vi "反控参数设置.vi"(8 "value time":timestamp, 9 "value float":sgl, 10 "设置参数":T2(ring)=enum."CODMn", 11 "设置类型":T1(ring)=enum."i13002") -> ()   [LabVIEW 2016]
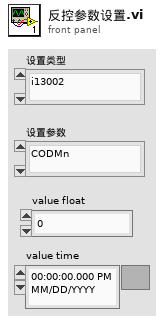
[diagram p1: front panel]
types:
  T1 = enum16{"i13001", "i13002", "i13003", "i13004", "i13005", "i13006", "i13007", "i13008", "i13009", "i13010", "i13011", "i13012", "i13013", "i13014", "i13015", "i13016", "i13017", "i13101", "i13102", "i13103", "i13104", "i13105", "i13106", "i13107", "i13108", "i13109", "i13110"}
  T2 = enum16{"", "CODMn", "PH", "氨氮", "总氮", "总磷", "CODCr", "电导率", "水温", "溶解氧", "浊度", "叶绿素", "藻密度", "ORP"}
  T3 = cluster{"status":bool, "代码":u16, "source":string}
  T4 = cluster{"测量量程":dbl, "测量精度":dbl, "测量间隔":dbl, "消解温度":dbl, "消解时长":dbl, "空白校准时间":timestamp, "曲线截距":dbl, "曲线斜率":dbl, "测量检出限":dbl, "测量信号值":dbl, "线性相关系数":dbl, "二次多项式系数":dbl, "标样校准时间":timestamp, "稀释倍数":dbl, "三项式系数":dbl, "空白标定系数":dbl, "量程系数":dbl, "F0/ORPA":dbl, "F1/ORPB":dbl, "F2/ORPK":dbl, "F3":dbl, "F4":dbl, "F5":dbl, "F6":dbl, "F7":dbl, "X0/滴定数":dbl, "量程":dbl}
  T5 = cluster{"测量量程":dbl, "测量精度":dbl, "测量间隔":dbl, "消解温度":dbl, "消解时长":dbl, "空白校准时间":timestamp, "曲线截距":dbl, "曲线斜率":dbl, "测量检出限":dbl, "测量信号值":dbl, "线性相关系数":dbl, "二次多项式系数":dbl, "标样校准时间":timestamp, "单位":u16}
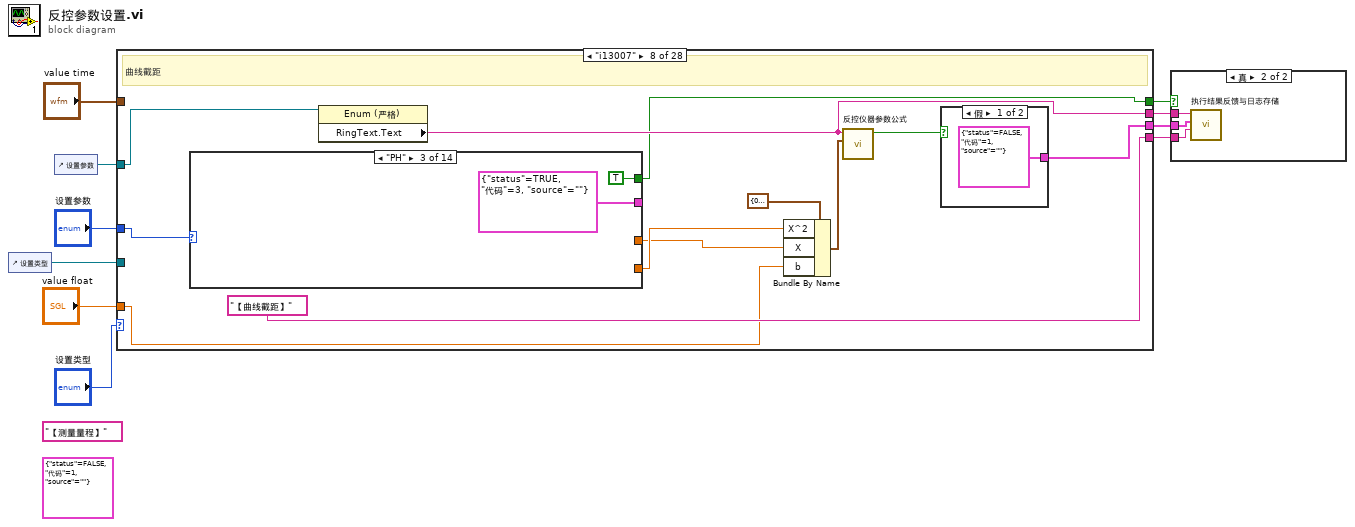
[diagram p0: block diagram]
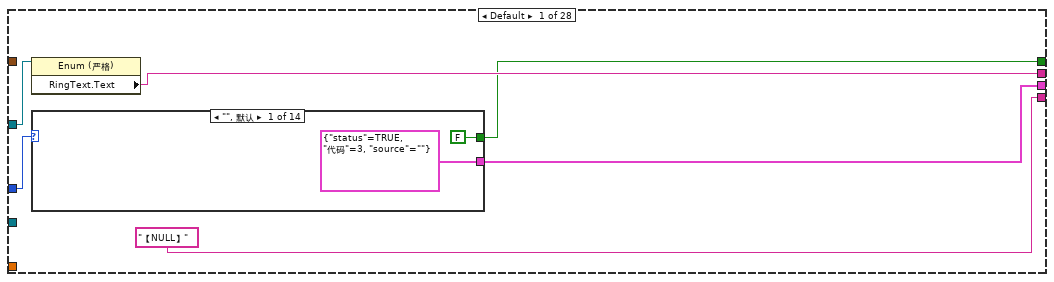
[diagram p3: hidden frame]
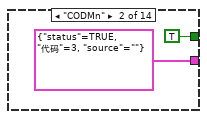
[diagram p4: hidden frame]
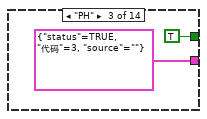
[diagram p5: hidden frame]
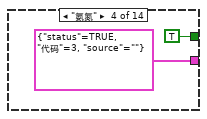
[diagram p6: hidden frame]
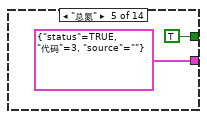
[diagram p7: hidden frame]
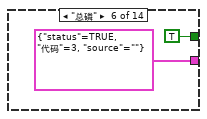
[diagram p8: hidden frame]
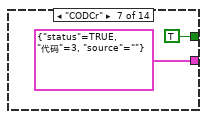
[diagram p9: hidden frame]
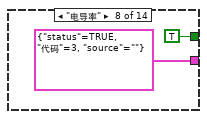
[diagram p10: hidden frame]
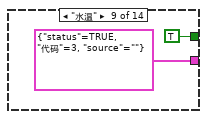
[diagram p11: hidden frame]
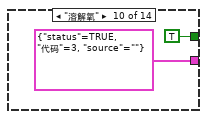
[diagram p12: hidden frame]
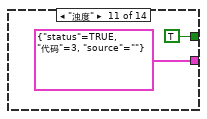
[diagram p13: hidden frame]
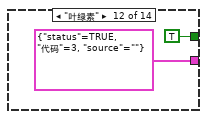
[diagram p14: hidden frame]
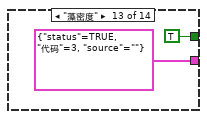
[diagram p15: hidden frame]
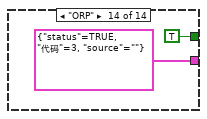
[diagram p16: hidden frame]
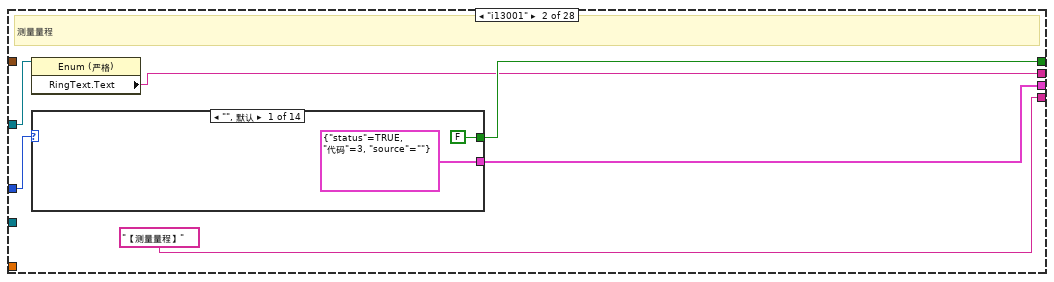
[diagram p17: hidden frame]
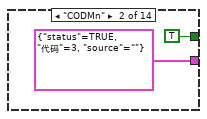
[diagram p18: hidden frame]
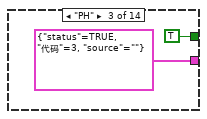
[diagram p19: hidden frame]
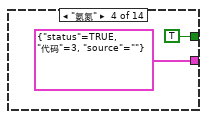
[diagram p20: hidden frame]
diagram:
  (unwired) T3 {"status"=FALSE, "代码"=1, "source"=""} ("error out")
  (unwired) "【测量量程】" ("日志信息")
  n1 = control-ref of="设置类型"() -> (w1:refnum<vi>)
  n2 = control-ref of="设置参数"() -> (w7:refnum<vi>)
  n3 = case shown="\"i13007\"" "设置类型" {
    tunnel: "设置参数" -> [w16 w50 w83 w114 w150 w193 w233 w270 w326 w381 w416 w452 w491 w540 w574 w608 w642 w676 w710 w744 w778 w816 w846 w880 w914 w948 w982 w1016]
    tunnel: [w12 w49 w80 w116 w152 w196 w236 w269 w327 w384 w418 w450 w494 w543 w577 w611 w645 w679 w713 w747 w781 w813 w849 w883 w917 w951 w985 w1019] -> w8
    tunnel: w7 -> [w15 w46 w84 w113 w154 w194 w234 w277 w334 w382 w415 w453 w492 w541 w575 w609 w643 w677 w711 w745 w779 w817 w847 w881 w915 w949 w983 w1017]
    tunnel: [w14 w45 w82 w118 w149 w190 w238 w273 w328 w386 w420 w454 w485 w545 w579 w613 w647 w681 w715 w749 w783 w815 w851 w885 w919 w953 w987 w1021] -> w6
    tunnel: ["【NULL】" ("日志信息") "【测量量程】" ("日志信息") "【测量精度】" ("日志信息") "【测量间隔】" ("日志信息") "【消解温度】" ("日志信息") "【消解时间】" ("日志信息") "【空白校准时间】" ("日志信息") "【曲线截距】" ("日志信息") "【曲线斜率】" ("日志信息") "【测量检出限】" ("日志信息") "【测量信号值】" ("日志信息") "【线性相关系数】" ("日志信息") "【二次项系数】" ("日志信息") "【标样校准时间】" ("日志信息") "【稀释倍数】" ("日志信息") "【三项式系数】" ("日志信息") "【空白标定系数】" ("日志信息") "【量程系数】" ("日志信息") "【F0/ORPA】" ("日志信息") "【F1/ORPB】" ("日志信息") "【F2/ORPK】" ("日志信息") "【F3】" ("日志信息") "【F4】" ("日志信息") "【F5】" ("日志信息") "【F6】" ("日志信息") "【F7】" ("日志信息") "【X0/滴定数】" ("日志信息") "【量程】" ("日志信息")] -> w5
    tunnel: [w13 w47 w81 w117 w153 w197 w237 w271 w330 w385 w419 w451 w487 w544 w578 w612 w646 w680 w714 w748 w782 w814 w850 w884 w918 w952 w986 w1020] -> w4
    tunnel: "value float" -> [_ _ _ _ w148 w192 _ w274 w329 _ _ _ w486 _ _ _ _ _ _ _ _ _ _ _ _ _ _ _]
    tunnel: "value time" -> [_ _ _ _ _ _ _ _ _ _ _ _ _ _ _ _ _ _ _ _ _ _ _ _ _ _ _ _]
    tunnel: w1 -> [_ _ _ _ w147 w191 _ _ _ _ _ _ _ _ _ _ _ _ _ _ _ _ _ _ _ _ _ _]
    frame Default {
      n4 = property class="Enum (严格)"(reference=w15) -> ("RingText.Text"=w14:string)  [unwired: 1 in, 2 out]
      n5 = case shown="\"\", 默认" w16 {
        tunnel: [FALSE TRUE TRUE TRUE TRUE TRUE TRUE TRUE TRUE TRUE TRUE TRUE TRUE TRUE] -> w12
        tunnel: [T3 {"status"=TRUE, "代码"=3, "source"=""} ("error out") T3 {"status"=TRUE, "代码"=3, "source"=""} ("error out") T3 {"status"=TRUE, "代码"=3, "source"=""} ("error out") T3 {"status"=TRUE, "代码"=3, "source"=""} ("error out") T3 {"status"=TRUE, "代码"=3, "source"=""} ("error out") T3 {"status"=TRUE, "代码"=3, "source"=""} ("error out") T3 {"status"=TRUE, "代码"=3, "source"=""} ("error out") T3 {"status"=TRUE, "代码"=3, "source"=""} ("error out") T3 {"status"=TRUE, "代码"=3, "source"=""} ("error out") T3 {"status"=TRUE, "代码"=3, "source"=""} ("error out") T3 {"status"=TRUE, "代码"=3, "source"=""} ("error out") T3 {"status"=TRUE, "代码"=3, "source"=""} ("error out") T3 {"status"=TRUE, "代码"=3, "source"=""} ("error out") T3 {"status"=TRUE, "代码"=3, "source"=""} ("error out")] -> w13
        frame "", Default {
        }
        frame "CODMn" {
        }
        frame "PH" {
        }
        frame "氨氮" {
        }
        frame "总氮" {
        }
        frame "总磷" {
        }
        frame "CODCr" {
        }
        frame "电导率" {
        }
        frame "水温" {
        }
        frame "溶解氧" {
        }
        frame "浊度" {
        }
        frame "叶绿素" {
        }
        frame "藻密度" {
        }
        frame "ORP" {
        }
      }
    }
    frame "i13001" {
      # "测量量程"
      n6 = property class="Enum (严格)"(reference=w46) -> ("RingText.Text"=w45:string)  [unwired: 1 in, 2 out]
      n7 = case shown="\"\", 默认" w50 {
        tunnel: [FALSE TRUE TRUE TRUE TRUE TRUE TRUE TRUE TRUE TRUE TRUE TRUE TRUE TRUE] -> w49
        tunnel: [T3 {"status"=TRUE, "代码"=3, "source"=""} ("error out") T3 {"status"=TRUE, "代码"=3, "source"=""} ("error out") T3 {"status"=TRUE, "代码"=3, "source"=""} ("error out") T3 {"status"=TRUE, "代码"=3, "source"=""} ("error out") T3 {"status"=TRUE, "代码"=3, "source"=""} ("error out") T3 {"status"=TRUE, "代码"=3, "source"=""} ("error out") T3 {"status"=TRUE, "代码"=3, "source"=""} ("error out") T3 {"status"=TRUE, "代码"=3, "source"=""} ("error out") T3 {"status"=TRUE, "代码"=3, "source"=""} ("error out") T3 {"status"=TRUE, "代码"=3, "source"=""} ("error out") T3 {"status"=TRUE, "代码"=3, "source"=""} ("error out") T3 {"status"=TRUE, "代码"=3, "source"=""} ("error out") T3 {"status"=TRUE, "代码"=3, "source"=""} ("error out") T3 {"status"=TRUE, "代码"=3, "source"=""} ("error out")] -> w47
        frame "", Default {
        }
        frame "CODMn" {
        }
        frame "PH" {
        }
        frame "氨氮" {
        }
        frame "总氮" {
        }
        frame "总磷" {
        }
        frame "CODCr" {
        }
        frame "电导率" {
        }
        frame "水温" {
        }
        frame "溶解氧" {
        }
        frame "浊度" {
        }
        frame "叶绿素" {
        }
        frame "藻密度" {
        }
        frame "ORP" {
        }
      }
    }
    frame "i13002" {
      # "测量精度"
      n8 = property class="Enum (严格)"(reference=w84) -> ("RingText.Text"=w82:string)  [unwired: 1 in, 2 out]
      n9 = case shown="\"\", 默认" w83 {
        tunnel: [FALSE TRUE TRUE TRUE TRUE TRUE TRUE TRUE TRUE TRUE TRUE TRUE TRUE TRUE] -> w80
        tunnel: [T3 {"status"=TRUE, "代码"=3, "source"=""} ("error out") T3 {"status"=TRUE, "代码"=3, "source"=""} ("error out") T3 {"status"=TRUE, "代码"=3, "source"=""} ("error out") T3 {"status"=TRUE, "代码"=3, "source"=""} ("error out") T3 {"status"=TRUE, "代码"=3, "source"=""} ("error out") T3 {"status"=TRUE, "代码"=3, "source"=""} ("error out") T3 {"status"=TRUE, "代码"=3, "source"=""} ("error out") T3 {"status"=TRUE, "代码"=3, "source"=""} ("error out") T3 {"status"=TRUE, "代码"=3, "source"=""} ("error out") T3 {"status"=TRUE, "代码"=3, "source"=""} ("error out") T3 {"status"=TRUE, "代码"=3, "source"=""} ("error out") T3 {"status"=TRUE, "代码"=3, "source"=""} ("error out") T3 {"status"=TRUE, "代码"=3, "source"=""} ("error out") T3 {"status"=TRUE, "代码"=3, "source"=""} ("error out")] -> w81
        frame "", Default {
        }
        frame "CODMn" {
        }
        frame "PH" {
        }
        frame "氨氮" {
        }
        frame "总氮" {
        }
        frame "总磷" {
        }
        frame "CODCr" {
        }
        frame "电导率" {
        }
        frame "水温" {
        }
        frame "溶解氧" {
        }
        frame "浊度" {
        }
        frame "叶绿素" {
        }
        frame "藻密度" {
        }
        frame "ORP" {
        }
      }
    }
    frame "i13003" {
      # "测量间隔"
      n10 = property class="Enum (严格)"(reference=w113) -> ("RingText.Text"=w118:string)  [unwired: 1 in, 2 out]
      n11 = case shown="\"\", 默认" w114 {
        tunnel: [FALSE TRUE TRUE TRUE TRUE TRUE TRUE TRUE TRUE TRUE TRUE TRUE TRUE TRUE] -> w116
        tunnel: [T3 {"status"=TRUE, "代码"=3, "source"=""} ("error out") T3 {"status"=TRUE, "代码"=3, "source"=""} ("error out") T3 {"status"=TRUE, "代码"=3, "source"=""} ("error out") T3 {"status"=TRUE, "代码"=3, "source"=""} ("error out") T3 {"status"=TRUE, "代码"=3, "source"=""} ("error out") T3 {"status"=TRUE, "代码"=3, "source"=""} ("error out") T3 {"status"=TRUE, "代码"=3, "source"=""} ("error out") T3 {"status"=TRUE, "代码"=3, "source"=""} ("error out") T3 {"status"=TRUE, "代码"=3, "source"=""} ("error out") T3 {"status"=TRUE, "代码"=3, "source"=""} ("error out") T3 {"status"=TRUE, "代码"=3, "source"=""} ("error out") T3 {"status"=TRUE, "代码"=3, "source"=""} ("error out") T3 {"status"=TRUE, "代码"=3, "source"=""} ("error out") T3 {"status"=TRUE, "代码"=3, "source"=""} ("error out")] -> w117
        frame "", Default {
        }
        frame "CODMn" {
        }
        frame "PH" {
        }
        frame "氨氮" {
        }
        frame "总氮" {
        }
        frame "总磷" {
        }
        frame "CODCr" {
        }
        frame "电导率" {
        }
        frame "水温" {
        }
        frame "溶解氧" {
        }
        frame "浊度" {
        }
        frame "叶绿素" {
        }
        frame "藻密度" {
        }
        frame "ORP" {
        }
      }
    }
    frame "i13004" {
      # "消解温度"
      n12 = property class="Enum (严格)"(reference=w154) -> ("RingText.Text"=w149:string)  [unwired: 1 in, 2 out]
      n13 = case shown="\"CODMn\"" w150 {
        tunnel: [FALSE TRUE TRUE TRUE TRUE TRUE TRUE TRUE TRUE TRUE TRUE TRUE TRUE TRUE] -> w152
        tunnel: [T3 {"status"=TRUE, "代码"=3, "source"=""} ("error out") w159 T3 {"status"=TRUE, "代码"=3, "source"=""} ("error out") T3 {"status"=TRUE, "代码"=3, "source"=""} ("error out") T3 {"status"=TRUE, "代码"=3, "source"=""} ("error out") T3 {"status"=TRUE, "代码"=3, "source"=""} ("error out") T3 {"status"=TRUE, "代码"=3, "source"=""} ("error out") T3 {"status"=TRUE, "代码"=3, "source"=""} ("error out") T3 {"status"=TRUE, "代码"=3, "source"=""} ("error out") T3 {"status"=TRUE, "代码"=3, "source"=""} ("error out") T3 {"status"=TRUE, "代码"=3, "source"=""} ("error out") T3 {"status"=TRUE, "代码"=3, "source"=""} ("error out") T3 {"status"=TRUE, "代码"=3, "source"=""} ("error out") T3 {"status"=TRUE, "代码"=3, "source"=""} ("error out")] -> w153
        tunnel: w149 -> [_ w162 _ _ _ _ _ _ _ _ _ _ _ _]
        tunnel: w148 -> [_ w161 _ _ _ _ _ _ _ _ _ _ _ _]
        tunnel: w147 -> [_ w158 _ _ _ _ _ _ _ _ _ _ _ _]
        frame "", Default {
        }
        frame "CODMn" {
          n14 = property class="Enum (严格)"(reference=w158) -> ("RingText.Text"=w157:string)  [unwired: 1 in, 2 out]
          n15 = call "反控仪器单参数通用.vi"("参数"=w162, "value float"=w161, "chose"=w157) -> ("超时？"=w160:bool)  [unwired: 7 in, 1 out]
          n16 = case shown="假" w160 {
            tunnel: [T3 {"status"=FALSE, "代码"=1, "source"=""} ("error out") T3 {"status"=TRUE, "代码"=4, "source"=""} ("error out")] -> w159
            frame False {
            }
            frame True {
            }
          }
        }
        frame "PH" {
        }
        frame "氨氮" {
        }
        frame "总氮" {
        }
        frame "总磷" {
        }
        frame "CODCr" {
        }
        frame "电导率" {
        }
        frame "水温" {
        }
        frame "溶解氧" {
        }
        frame "浊度" {
        }
        frame "叶绿素" {
        }
        frame "藻密度" {
        }
        frame "ORP" {
        }
      }
    }
    frame "i13005" {
      # "消解时间"
      n17 = property class="Enum (严格)"(reference=w194) -> ("RingText.Text"=w190:string)  [unwired: 1 in, 2 out]
      n18 = case shown="\"CODMn\"" w193 {
        tunnel: [FALSE TRUE TRUE TRUE TRUE TRUE TRUE TRUE TRUE TRUE TRUE TRUE TRUE TRUE] -> w196
        tunnel: [T3 {"status"=TRUE, "代码"=3, "source"=""} ("error out") w200 T3 {"status"=TRUE, "代码"=3, "source"=""} ("error out") T3 {"status"=TRUE, "代码"=3, "source"=""} ("error out") T3 {"status"=TRUE, "代码"=3, "source"=""} ("error out") T3 {"status"=TRUE, "代码"=3, "source"=""} ("error out") T3 {"status"=TRUE, "代码"=3, "source"=""} ("error out") T3 {"status"=TRUE, "代码"=3, "source"=""} ("error out") T3 {"status"=TRUE, "代码"=3, "source"=""} ("error out") T3 {"status"=TRUE, "代码"=3, "source"=""} ("error out") T3 {"status"=TRUE, "代码"=3, "source"=""} ("error out") T3 {"status"=TRUE, "代码"=3, "source"=""} ("error out") T3 {"status"=TRUE, "代码"=3, "source"=""} ("error out") T3 {"status"=TRUE, "代码"=3, "source"=""} ("error out")] -> w197
        tunnel: w192 -> [_ w203 _ _ _ _ _ _ _ _ _ _ _ _]
        tunnel: w191 -> [_ w202 _ _ _ _ _ _ _ _ _ _ _ _]
        tunnel: w190 -> [_ w201 _ _ _ _ _ _ _ _ _ _ _ _]
        frame "", Default {
        }
        frame "CODMn" {
          n19 = property class="Enum (严格)"(reference=w202) -> ("RingText.Text"=w204:string)  [unwired: 1 in, 2 out]
          n20 = call "反控仪器单参数通用.vi"("参数"=w201, "value float"=w203, "chose"=w204) -> ("超时？"=w205:bool)  [unwired: 7 in, 1 out]
          n21 = case shown="假" w205 {
            tunnel: [T3 {"status"=FALSE, "代码"=1, "source"=""} ("error out") T3 {"status"=TRUE, "代码"=4, "source"=""} ("error out")] -> w200
            frame False {
            }
            frame True {
            }
          }
        }
        frame "PH" {
        }
        frame "氨氮" {
        }
        frame "总氮" {
        }
        frame "总磷" {
        }
        frame "CODCr" {
        }
        frame "电导率" {
        }
        frame "水温" {
        }
        frame "溶解氧" {
        }
        frame "浊度" {
        }
        frame "叶绿素" {
        }
        frame "藻密度" {
        }
        frame "ORP" {
        }
      }
    }
    frame "i13006" {
      # "空白校准时间"
      n22 = property class="Enum (严格)"(reference=w234) -> ("RingText.Text"=w238:string)  [unwired: 1 in, 2 out]
      n23 = case shown="\"电导率\"" w233 {
        tunnel: [FALSE TRUE TRUE TRUE TRUE TRUE TRUE TRUE TRUE TRUE TRUE TRUE TRUE TRUE] -> w236
        tunnel: [T3 {"status"=TRUE, "代码"=3, "source"=""} ("error out") T3 {"status"=TRUE, "代码"=3, "source"=""} ("error out") T3 {"status"=TRUE, "代码"=3, "source"=""} ("error out") T3 {"status"=TRUE, "代码"=3, "source"=""} ("error out") T3 {"status"=TRUE, "代码"=3, "source"=""} ("error out") T3 {"status"=TRUE, "代码"=3, "source"=""} ("error out") T3 {"status"=TRUE, "代码"=3, "source"=""} ("error out") T3 {"status"=TRUE, "代码"=3, "source"=""} ("error out") T3 {"status"=TRUE, "代码"=3, "source"=""} ("error out") T3 {"status"=TRUE, "代码"=3, "source"=""} ("error out") T3 {"status"=TRUE, "代码"=3, "source"=""} ("error out") T3 {"status"=TRUE, "代码"=3, "source"=""} ("error out") T3 {"status"=TRUE, "代码"=3, "source"=""} ("error out") T3 {"status"=TRUE, "代码"=3, "source"=""} ("error out")] -> w237
        frame "", Default {
        }
        frame "CODMn" {
        }
        frame "PH" {
        }
        frame "氨氮" {
        }
        frame "总氮" {
        }
        frame "总磷" {
        }
        frame "CODCr" {
        }
        frame "电导率" {
        }
        frame "水温" {
        }
        frame "溶解氧" {
        }
        frame "浊度" {
        }
        frame "叶绿素" {
        }
        frame "藻密度" {
        }
        frame "ORP" {
        }
      }
    }
    frame "i13007" {
      # "曲线截距"
      n24 = case shown="\"PH\"" w270 {
        tunnel: [FALSE TRUE TRUE TRUE TRUE TRUE TRUE TRUE TRUE TRUE TRUE TRUE TRUE TRUE] -> w269
        tunnel: [T3 {"status"=TRUE, "代码"=3, "source"=""} ("error out") T3 {"status"=TRUE, "代码"=3, "source"=""} ("error out") T3 {"status"=TRUE, "代码"=3, "source"=""} ("error out") T3 {"status"=TRUE, "代码"=3, "source"=""} ("error out") T3 {"status"=TRUE, "代码"=3, "source"=""} ("error out") T3 {"status"=TRUE, "代码"=3, "source"=""} ("error out") T3 {"status"=TRUE, "代码"=3, "source"=""} ("error out") T3 {"status"=TRUE, "代码"=3, "source"=""} ("error out") T3 {"status"=TRUE, "代码"=3, "source"=""} ("error out") T3 {"status"=TRUE, "代码"=3, "source"=""} ("error out") T3 {"status"=TRUE, "代码"=3, "source"=""} ("error out") T3 {"status"=TRUE, "代码"=3, "source"=""} ("error out") T3 {"status"=TRUE, "代码"=3, "source"=""} ("error out") T3 {"status"=TRUE, "代码"=3, "source"=""} ("error out")] -> _
        tunnel: [_ w282 _ w289 w294 w299 w304 _ _ _ _ _ _ _] -> w267
        tunnel: [_ w281 _ w288 w293 w298 w303 _ _ _ _ _ _ _] -> w268
        frame "", Default {
        }
        frame "CODMn" {
          n25 = global read "CODMn断电保存全局变量.vi" "CODMn仪器参数"() -> (w283:T4)
          n26 = Unbundle By Name(w283) -> ("曲线斜率"=w282:dbl, "二次多项式系数"=w281:dbl)
        }
        frame "PH" {
        }
        frame "氨氮" {
          n27 = global read "氨氮断电保存全局变量.vi" "氨氮仪器参数"() -> (w290:T4)
          n28 = Unbundle By Name(w290) -> ("曲线斜率"=w289:dbl, "二次多项式系数"=w288:dbl)
        }
        frame "总氮" {
          n29 = global read "总氮断电保存全局变量.vi" "总氮仪器参数"() -> (w295:T5)
          n30 = Unbundle By Name(w295) -> ("曲线斜率"=w294:dbl, "二次多项式系数"=w293:dbl)
        }
        frame "总磷" {
          n31 = global read "总磷断电保存全局变量.vi" "总磷仪器参数"() -> (w300:T5)
          n32 = Unbundle By Name(w300) -> ("曲线斜率"=w299:dbl, "二次多项式系数"=w298:dbl)
        }
        frame "CODCr" {
          n33 = global read "CODcr全局变量.vi" "CODCr仪器参数"() -> (w305:T4)
          n34 = Unbundle By Name(w305) -> ("曲线斜率"=w304:dbl, "二次多项式系数"=w303:dbl)
        }
        frame "电导率" {
        }
        frame "水温" {
        }
        frame "溶解氧" {
        }
        frame "浊度" {
        }
        frame "叶绿素" {
        }
        frame "藻密度" {
        }
        frame "ORP" {
        }
      }
      n35 = property class="Enum (严格)"(reference=w277) -> ("RingText.Text"=w273:string)  [unwired: 1 in, 2 out]
      n36 = Bundle By Name(cluster=cluster{"X^2":dbl, "X":dbl, "b":dbl} {"X^2"=0.0, "X"=0.0, "b"=0.0} ("公式"), "X^2"=w268, "X"=w267, "b"=w274) -> (w276:cluster{"X^2":dbl, "X":dbl, "b":dbl})
      n37 = call "反控仪器参数公式.vi"("公式"=w276, "参数"=w273) -> ("超时？"=w272:bool)  [unwired: 8 in, 1 out]
      n38 = case shown="假" w272 {
        tunnel: [T3 {"status"=FALSE, "代码"=1, "source"=""} ("error out") T3 {"status"=TRUE, "代码"=4, "source"=""} ("error out")] -> w271
        frame False {
        }
        frame True {
        }
      }
    }
    frame "i13008" {
      # "曲线斜率"
      n39 = case shown="\"电导率\"" w326 {
        tunnel: [FALSE TRUE TRUE TRUE TRUE TRUE TRUE TRUE TRUE TRUE TRUE TRUE TRUE TRUE] -> w327
        tunnel: [T3 {"status"=TRUE, "代码"=3, "source"=""} ("error out") T3 {"status"=TRUE, "代码"=3, "source"=""} ("error out") T3 {"status"=TRUE, "代码"=3, "source"=""} ("error out") T3 {"status"=TRUE, "代码"=3, "source"=""} ("error out") T3 {"status"=TRUE, "代码"=3, "source"=""} ("error out") T3 {"status"=TRUE, "代码"=3, "source"=""} ("error out") T3 {"status"=TRUE, "代码"=3, "source"=""} ("error out") T3 {"status"=TRUE, "代码"=3, "source"=""} ("error out") T3 {"status"=TRUE, "代码"=3, "source"=""} ("error out") T3 {"status"=TRUE, "代码"=3, "source"=""} ("error out") T3 {"status"=TRUE, "代码"=3, "source"=""} ("error out") T3 {"status"=TRUE, "代码"=3, "source"=""} ("error out") T3 {"status"=TRUE, "代码"=3, "source"=""} ("error out") T3 {"status"=TRUE, "代码"=3, "source"=""} ("error out")] -> _
        tunnel: [_ w339 _ w346 w351 w356 w361 _ _ _ _ _ _ _] -> w325
        tunnel: [_ w338 _ w345 w350 w355 w360 _ _ _ _ _ _ _] -> w324
        frame "", Default {
        }
        frame "CODMn" {
          n40 = global read "CODMn断电保存全局变量.vi" "CODMn仪器参数"() -> (w340:T4)
          n41 = Unbundle By Name(w340) -> ("曲线截距"=w339:dbl, "二次多项式系数"=w338:dbl)
        }
        frame "PH" {
        }
        frame "氨氮" {
          n42 = global read "氨氮断电保存全局变量.vi" "氨氮仪器参数"() -> (w347:T4)
          n43 = Unbundle By Name(w347) -> ("曲线截距"=w346:dbl, "二次多项式系数"=w345:dbl)
        }
        frame "总氮" {
          n44 = global read "总氮断电保存全局变量.vi" "总氮仪器参数"() -> (w352:T5)
          n45 = Unbundle By Name(w352) -> ("曲线截距"=w351:dbl, "二次多项式系数"=w350:dbl)
        }
        frame "总磷" {
          n46 = global read "总磷断电保存全局变量.vi" "总磷仪器参数"() -> (w357:T5)
          n47 = Unbundle By Name(w357) -> ("曲线截距"=w356:dbl, "二次多项式系数"=w355:dbl)
        }
        frame "CODCr" {
          n48 = global read "CODcr全局变量.vi" "CODCr仪器参数"() -> (w362:T4)
          n49 = Unbundle By Name(w362) -> ("曲线截距"=w361:dbl, "二次多项式系数"=w360:dbl)
        }
        frame "电导率" {
        }
        frame "水温" {
        }
        frame "溶解氧" {
        }
        frame "浊度" {
        }
        frame "叶绿素" {
        }
        frame "藻密度" {
        }
        frame "ORP" {
        }
      }
      n50 = property class="Enum (严格)"(reference=w334) -> ("RingText.Text"=w328:string)  [unwired: 1 in, 2 out]
      n51 = Bundle By Name(cluster=cluster{"X^2":dbl, "X":dbl, "b":dbl} {"X^2"=0.0, "X"=0.0, "b"=0.0} ("公式"), "X^2"=w324, "X"=w329, "b"=w325) -> (w331:cluster{"X^2":dbl, "X":dbl, "b":dbl})
      n52 = call "反控仪器参数公式.vi"("公式"=w331, "参数"=w328) -> ("超时？"=w333:bool)  [unwired: 8 in, 1 out]
      n53 = case shown="假" w333 {
        tunnel: [T3 {"status"=FALSE, "代码"=1, "source"=""} ("error out") T3 {"status"=TRUE, "代码"=4, "source"=""} ("error out")] -> w330
        frame False {
        }
        frame True {
        }
      }
    }
    frame "i13009" {
      # "测量检出限"
      n54 = property class="Enum (严格)"(reference=w382) -> ("RingText.Text"=w386:string)  [unwired: 1 in, 2 out]
      n55 = case shown="\"\", 默认" w381 {
        tunnel: [FALSE TRUE TRUE TRUE TRUE TRUE TRUE TRUE TRUE TRUE TRUE TRUE TRUE TRUE] -> w384
        tunnel: [T3 {"status"=TRUE, "代码"=3, "source"=""} ("error out") T3 {"status"=TRUE, "代码"=3, "source"=""} ("error out") T3 {"status"=TRUE, "代码"=3, "source"=""} ("error out") T3 {"status"=TRUE, "代码"=3, "source"=""} ("error out") T3 {"status"=TRUE, "代码"=3, "source"=""} ("error out") T3 {"status"=TRUE, "代码"=3, "source"=""} ("error out") T3 {"status"=TRUE, "代码"=3, "source"=""} ("error out") T3 {"status"=TRUE, "代码"=3, "source"=""} ("error out") T3 {"status"=TRUE, "代码"=3, "source"=""} ("error out") T3 {"status"=TRUE, "代码"=3, "source"=""} ("error out") T3 {"status"=TRUE, "代码"=3, "source"=""} ("error out") T3 {"status"=TRUE, "代码"=3, "source"=""} ("error out") T3 {"status"=TRUE, "代码"=3, "source"=""} ("error out") T3 {"status"=TRUE, "代码"=3, "source"=""} ("error out")] -> w385
        frame "", Default {
        }
        frame "CODMn" {
        }
        frame "PH" {
        }
        frame "氨氮" {
        }
        frame "总氮" {
        }
        frame "总磷" {
        }
        frame "CODCr" {
        }
        frame "电导率" {
        }
        frame "水温" {
        }
        frame "溶解氧" {
        }
        frame "浊度" {
        }
        frame "叶绿素" {
        }
        frame "藻密度" {
        }
        frame "ORP" {
        }
      }
    }
    frame "i13010" {
      # "测量信号值"
      n56 = property class="Enum (严格)"(reference=w415) -> ("RingText.Text"=w420:string)  [unwired: 1 in, 2 out]
      n57 = case shown="\"浊度\"" w416 {
        tunnel: [FALSE TRUE TRUE TRUE TRUE TRUE TRUE TRUE TRUE TRUE TRUE TRUE TRUE TRUE] -> w418
        tunnel: [T3 {"status"=TRUE, "代码"=3, "source"=""} ("error out") T3 {"status"=TRUE, "代码"=3, "source"=""} ("error out") T3 {"status"=TRUE, "代码"=3, "source"=""} ("error out") T3 {"status"=TRUE, "代码"=3, "source"=""} ("error out") T3 {"status"=TRUE, "代码"=3, "source"=""} ("error out") T3 {"status"=TRUE, "代码"=3, "source"=""} ("error out") T3 {"status"=TRUE, "代码"=3, "source"=""} ("error out") T3 {"status"=TRUE, "代码"=3, "source"=""} ("error out") T3 {"status"=TRUE, "代码"=3, "source"=""} ("error out") T3 {"status"=TRUE, "代码"=3, "source"=""} ("error out") T3 {"status"=TRUE, "代码"=3, "source"=""} ("error out") T3 {"status"=TRUE, "代码"=3, "source"=""} ("error out") T3 {"status"=TRUE, "代码"=3, "source"=""} ("error out") T3 {"status"=TRUE, "代码"=3, "source"=""} ("error out")] -> w419
        frame "", Default {
        }
        frame "CODMn" {
        }
        frame "PH" {
        }
        frame "氨氮" {
        }
        frame "总氮" {
        }
        frame "总磷" {
        }
        frame "CODCr" {
        }
        frame "电导率" {
        }
        frame "水温" {
        }
        frame "溶解氧" {
        }
        frame "浊度" {
        }
        frame "叶绿素" {
        }
        frame "藻密度" {
        }
        frame "ORP" {
        }
      }
    }
    frame "i13011" {
      # "线性相关系数"
      n58 = property class="Enum (严格)"(reference=w453) -> ("RingText.Text"=w454:string)  [unwired: 1 in, 2 out]
      n59 = case shown="\"\", 默认" w452 {
        tunnel: [FALSE TRUE TRUE TRUE TRUE TRUE TRUE TRUE TRUE TRUE TRUE TRUE TRUE TRUE] -> w450
        tunnel: [T3 {"status"=TRUE, "代码"=3, "source"=""} ("error out") T3 {"status"=TRUE, "代码"=3, "source"=""} ("error out") T3 {"status"=TRUE, "代码"=3, "source"=""} ("error out") T3 {"status"=TRUE, "代码"=3, "source"=""} ("error out") T3 {"status"=TRUE, "代码"=3, "source"=""} ("error out") T3 {"status"=TRUE, "代码"=3, "source"=""} ("error out") T3 {"status"=TRUE, "代码"=3, "source"=""} ("error out") T3 {"status"=TRUE, "代码"=3, "source"=""} ("error out") T3 {"status"=TRUE, "代码"=3, "source"=""} ("error out") T3 {"status"=TRUE, "代码"=3, "source"=""} ("error out") T3 {"status"=TRUE, "代码"=3, "source"=""} ("error out") T3 {"status"=TRUE, "代码"=3, "source"=""} ("error out") T3 {"status"=TRUE, "代码"=3, "source"=""} ("error out") T3 {"status"=TRUE, "代码"=3, "source"=""} ("error out")] -> w451
        frame "", Default {
        }
        frame "CODMn" {
        }
        frame "PH" {
        }
        frame "氨氮" {
        }
        frame "总氮" {
        }
        frame "总磷" {
        }
        frame "CODCr" {
        }
        frame "电导率" {
        }
        frame "水温" {
        }
        frame "溶解氧" {
        }
        frame "浊度" {
        }
        frame "叶绿素" {
        }
        frame "藻密度" {
        }
        frame "ORP" {
        }
      }
    }
    frame "i13012" {
      # "二次项系数"
      n60 = case shown="\"PH\"" w491 {
        tunnel: [FALSE TRUE TRUE TRUE TRUE TRUE TRUE TRUE TRUE TRUE TRUE TRUE TRUE TRUE] -> w494
        tunnel: [T3 {"status"=TRUE, "代码"=3, "source"=""} ("error out") T3 {"status"=TRUE, "代码"=3, "source"=""} ("error out") T3 {"status"=TRUE, "代码"=3, "source"=""} ("error out") T3 {"status"=TRUE, "代码"=3, "source"=""} ("error out") T3 {"status"=TRUE, "代码"=3, "source"=""} ("error out") T3 {"status"=TRUE, "代码"=3, "source"=""} ("error out") T3 {"status"=TRUE, "代码"=3, "source"=""} ("error out") T3 {"status"=TRUE, "代码"=3, "source"=""} ("error out") T3 {"status"=TRUE, "代码"=3, "source"=""} ("error out") T3 {"status"=TRUE, "代码"=3, "source"=""} ("error out") T3 {"status"=TRUE, "代码"=3, "source"=""} ("error out") T3 {"status"=TRUE, "代码"=3, "source"=""} ("error out") T3 {"status"=TRUE, "代码"=3, "source"=""} ("error out") T3 {"status"=TRUE, "代码"=3, "source"=""} ("error out")] -> _
        tunnel: [_ w500 _ w507 w512 w517 w522 _ _ _ _ _ _ _] -> w484
        tunnel: [_ w499 _ w506 w511 w516 w521 _ _ _ _ _ _ _] -> w483
        frame "", Default {
        }
        frame "CODMn" {
          n61 = global read "CODMn断电保存全局变量.vi" "CODMn仪器参数"() -> (w501:T4)
          n62 = Unbundle By Name(w501) -> ("曲线截距"=w500:dbl, "曲线斜率"=w499:dbl)
        }
        frame "PH" {
        }
        frame "氨氮" {
          n63 = global read "氨氮断电保存全局变量.vi" "氨氮仪器参数"() -> (w508:T4)
          n64 = Unbundle By Name(w508) -> ("曲线截距"=w507:dbl, "曲线斜率"=w506:dbl)
        }
        frame "总氮" {
          n65 = global read "总氮断电保存全局变量.vi" "总氮仪器参数"() -> (w513:T5)
          n66 = Unbundle By Name(w513) -> ("曲线截距"=w512:dbl, "曲线斜率"=w511:dbl)
        }
        frame "总磷" {
          n67 = global read "总磷断电保存全局变量.vi" "总磷仪器参数"() -> (w518:T5)
          n68 = Unbundle By Name(w518) -> ("曲线截距"=w517:dbl, "曲线斜率"=w516:dbl)
        }
        frame "CODCr" {
          n69 = global read "CODcr全局变量.vi" "CODCr仪器参数"() -> (w523:T4)
          n70 = Unbundle By Name(w523) -> ("曲线截距"=w522:dbl, "曲线斜率"=w521:dbl)
        }
        frame "电导率" {
        }
        frame "水温" {
        }
        frame "溶解氧" {
        }
        frame "浊度" {
        }
        frame "叶绿素" {
        }
        frame "藻密度" {
        }
        frame "ORP" {
        }
      }
      n71 = property class="Enum (严格)"(reference=w492) -> ("RingText.Text"=w485:string)  [unwired: 1 in, 2 out]
      n72 = Bundle By Name(cluster=cluster{"X^2":dbl, "X":dbl, "b":dbl} {"X^2"=0.0, "X"=0.0, "b"=0.0} ("公式"), "X^2"=w486, "X"=w483, "b"=w484) -> (w488:cluster{"X^2":dbl, "X":dbl, "b":dbl})
      n73 = call "反控仪器参数公式.vi"("公式"=w488, "参数"=w485) -> ("超时？"=w490:bool)  [unwired: 8 in, 1 out]
      n74 = case shown="假" w490 {
        tunnel: [T3 {"status"=FALSE, "代码"=1, "source"=""} ("error out") T3 {"status"=TRUE, "代码"=4, "source"=""} ("error out")] -> w487
        frame False {
        }
        frame True {
        }
      }
    }
    frame "i13013" {
      # "标样校准时间"
      n75 = property class="Enum (严格)"(reference=w541) -> ("RingText.Text"=w545:string)  [unwired: 1 in, 2 out]
      n76 = case shown="\"CODMn\"" w540 {
        tunnel: [FALSE TRUE TRUE TRUE TRUE TRUE TRUE TRUE TRUE TRUE TRUE TRUE TRUE TRUE] -> w543
        tunnel: [T3 {"status"=TRUE, "代码"=3, "source"=""} ("error out") T3 {"status"=TRUE, "代码"=3, "source"=""} ("error out") T3 {"status"=TRUE, "代码"=3, "source"=""} ("error out") T3 {"status"=TRUE, "代码"=3, "source"=""} ("error out") T3 {"status"=TRUE, "代码"=3, "source"=""} ("error out") T3 {"status"=TRUE, "代码"=3, "source"=""} ("error out") T3 {"status"=TRUE, "代码"=3, "source"=""} ("error out") T3 {"status"=TRUE, "代码"=3, "source"=""} ("error out") T3 {"status"=TRUE, "代码"=3, "source"=""} ("error out") T3 {"status"=TRUE, "代码"=3, "source"=""} ("error out") T3 {"status"=TRUE, "代码"=3, "source"=""} ("error out") T3 {"status"=TRUE, "代码"=3, "source"=""} ("error out") T3 {"status"=TRUE, "代码"=3, "source"=""} ("error out") T3 {"status"=TRUE, "代码"=3, "source"=""} ("error out")] -> w544
        frame "", Default {
        }
        frame "CODMn" {
        }
        frame "PH" {
        }
        frame "氨氮" {
        }
        frame "总氮" {
        }
        frame "总磷" {
        }
        frame "CODCr" {
        }
        frame "电导率" {
        }
        frame "水温" {
        }
        frame "溶解氧" {
        }
        frame "浊度" {
        }
        frame "叶绿素" {
        }
        frame "藻密度" {
        }
        frame "ORP" {
        }
      }
    }
    frame "i13014" {
      # "稀释倍数"
      n77 = property class="Enum (严格)"(reference=w575) -> ("RingText.Text"=w579:string)  [unwired: 1 in, 2 out]
      n78 = case shown="\"\", 默认" w574 {
        tunnel: [FALSE TRUE TRUE TRUE TRUE TRUE TRUE TRUE TRUE TRUE TRUE TRUE TRUE TRUE] -> w577
        tunnel: [T3 {"status"=TRUE, "代码"=3, "source"=""} ("error out") T3 {"status"=TRUE, "代码"=3, "source"=""} ("error out") T3 {"status"=TRUE, "代码"=3, "source"=""} ("error out") T3 {"status"=TRUE, "代码"=3, "source"=""} ("error out") T3 {"status"=TRUE, "代码"=3, "source"=""} ("error out") T3 {"status"=TRUE, "代码"=3, "source"=""} ("error out") T3 {"status"=TRUE, "代码"=3, "source"=""} ("error out") T3 {"status"=TRUE, "代码"=3, "source"=""} ("error out") T3 {"status"=TRUE, "代码"=3, "source"=""} ("error out") T3 {"status"=TRUE, "代码"=3, "source"=""} ("error out") T3 {"status"=TRUE, "代码"=3, "source"=""} ("error out") T3 {"status"=TRUE, "代码"=3, "source"=""} ("error out") T3 {"status"=TRUE, "代码"=3, "source"=""} ("error out") T3 {"status"=TRUE, "代码"=3, "source"=""} ("error out")] -> w578
        frame "", Default {
        }
        frame "CODMn" {
        }
        frame "PH" {
        }
        frame "氨氮" {
        }
        frame "总氮" {
        }
        frame "总磷" {
        }
        frame "CODCr" {
        }
        frame "电导率" {
        }
        frame "水温" {
        }
        frame "溶解氧" {
        }
        frame "浊度" {
        }
        frame "叶绿素" {
        }
        frame "藻密度" {
        }
        frame "ORP" {
        }
      }
    }
    frame "i13015" {
      # "三项式系数"
      n79 = property class="Enum (严格)"(reference=w609) -> ("RingText.Text"=w613:string)  [unwired: 1 in, 2 out]
      n80 = case shown="\"\", 默认" w608 {
        tunnel: [FALSE TRUE TRUE TRUE TRUE TRUE TRUE TRUE TRUE TRUE TRUE TRUE TRUE TRUE] -> w611
        tunnel: [T3 {"status"=TRUE, "代码"=3, "source"=""} ("error out") T3 {"status"=TRUE, "代码"=3, "source"=""} ("error out") T3 {"status"=TRUE, "代码"=3, "source"=""} ("error out") T3 {"status"=TRUE, "代码"=3, "source"=""} ("error out") T3 {"status"=TRUE, "代码"=3, "source"=""} ("error out") T3 {"status"=TRUE, "代码"=3, "source"=""} ("error out") T3 {"status"=TRUE, "代码"=3, "source"=""} ("error out") T3 {"status"=TRUE, "代码"=3, "source"=""} ("error out") T3 {"status"=TRUE, "代码"=3, "source"=""} ("error out") T3 {"status"=TRUE, "代码"=3, "source"=""} ("error out") T3 {"status"=TRUE, "代码"=3, "source"=""} ("error out") T3 {"status"=TRUE, "代码"=3, "source"=""} ("error out") T3 {"status"=TRUE, "代码"=3, "source"=""} ("error out") T3 {"status"=TRUE, "代码"=3, "source"=""} ("error out")] -> w612
        frame "", Default {
        }
        frame "CODMn" {
        }
        frame "PH" {
        }
        frame "氨氮" {
        }
        frame "总氮" {
        }
        frame "总磷" {
        }
        frame "CODCr" {
        }
        frame "电导率" {
        }
        frame "水温" {
        }
        frame "溶解氧" {
        }
        frame "浊度" {
        }
        frame "叶绿素" {
        }
        frame "藻密度" {
        }
        frame "ORP" {
        }
      }
    }
    frame "i13016" {
      # "空白标定系数"
      n81 = property class="Enum (严格)"(reference=w643) -> ("RingText.Text"=w647:string)  [unwired: 1 in, 2 out]
      n82 = case shown="\"\", 默认" w642 {
        tunnel: [FALSE TRUE TRUE TRUE TRUE TRUE TRUE TRUE TRUE TRUE TRUE TRUE TRUE TRUE] -> w645
        tunnel: [T3 {"status"=TRUE, "代码"=3, "source"=""} ("error out") T3 {"status"=TRUE, "代码"=3, "source"=""} ("error out") T3 {"status"=TRUE, "代码"=3, "source"=""} ("error out") T3 {"status"=TRUE, "代码"=3, "source"=""} ("error out") T3 {"status"=TRUE, "代码"=3, "source"=""} ("error out") T3 {"status"=TRUE, "代码"=3, "source"=""} ("error out") T3 {"status"=TRUE, "代码"=3, "source"=""} ("error out") T3 {"status"=TRUE, "代码"=3, "source"=""} ("error out") T3 {"status"=TRUE, "代码"=3, "source"=""} ("error out") T3 {"status"=TRUE, "代码"=3, "source"=""} ("error out") T3 {"status"=TRUE, "代码"=3, "source"=""} ("error out") T3 {"status"=TRUE, "代码"=3, "source"=""} ("error out") T3 {"status"=TRUE, "代码"=3, "source"=""} ("error out") T3 {"status"=TRUE, "代码"=3, "source"=""} ("error out")] -> w646
        frame "", Default {
        }
        frame "CODMn" {
        }
        frame "PH" {
        }
        frame "氨氮" {
        }
        frame "总氮" {
        }
        frame "总磷" {
        }
        frame "CODCr" {
        }
        frame "电导率" {
        }
        frame "水温" {
        }
        frame "溶解氧" {
        }
        frame "浊度" {
        }
        frame "叶绿素" {
        }
        frame "藻密度" {
        }
        frame "ORP" {
        }
      }
    }
    frame "i13017" {
      # "量程系数"
      n83 = property class="Enum (严格)"(reference=w677) -> ("RingText.Text"=w681:string)  [unwired: 1 in, 2 out]
      n84 = case shown="\"\", 默认" w676 {
        tunnel: [FALSE TRUE TRUE TRUE TRUE TRUE TRUE TRUE TRUE TRUE TRUE TRUE TRUE TRUE] -> w679
        tunnel: [T3 {"status"=TRUE, "代码"=3, "source"=""} ("error out") T3 {"status"=TRUE, "代码"=3, "source"=""} ("error out") T3 {"status"=TRUE, "代码"=3, "source"=""} ("error out") T3 {"status"=TRUE, "代码"=3, "source"=""} ("error out") T3 {"status"=TRUE, "代码"=3, "source"=""} ("error out") T3 {"status"=TRUE, "代码"=3, "source"=""} ("error out") T3 {"status"=TRUE, "代码"=3, "source"=""} ("error out") T3 {"status"=TRUE, "代码"=3, "source"=""} ("error out") T3 {"status"=TRUE, "代码"=3, "source"=""} ("error out") T3 {"status"=TRUE, "代码"=3, "source"=""} ("error out") T3 {"status"=TRUE, "代码"=3, "source"=""} ("error out") T3 {"status"=TRUE, "代码"=3, "source"=""} ("error out") T3 {"status"=TRUE, "代码"=3, "source"=""} ("error out") T3 {"status"=TRUE, "代码"=3, "source"=""} ("error out")] -> w680
        frame "", Default {
        }
        frame "CODMn" {
        }
        frame "PH" {
        }
        frame "氨氮" {
        }
        frame "总氮" {
        }
        frame "总磷" {
        }
        frame "CODCr" {
        }
        frame "电导率" {
        }
        frame "水温" {
        }
        frame "溶解氧" {
        }
        frame "浊度" {
        }
        frame "叶绿素" {
        }
        frame "藻密度" {
        }
        frame "ORP" {
        }
      }
    }
    frame "i13101" {
      # "F0/ORPA"
      n85 = property class="Enum (严格)"(reference=w711) -> ("RingText.Text"=w715:string)  [unwired: 1 in, 2 out]
      n86 = case shown="\"\", 默认" w710 {
        tunnel: [FALSE TRUE TRUE TRUE TRUE TRUE TRUE TRUE TRUE TRUE TRUE TRUE TRUE TRUE] -> w713
        tunnel: [T3 {"status"=TRUE, "代码"=3, "source"=""} ("error out") T3 {"status"=TRUE, "代码"=3, "source"=""} ("error out") T3 {"status"=TRUE, "代码"=3, "source"=""} ("error out") T3 {"status"=TRUE, "代码"=3, "source"=""} ("error out") T3 {"status"=TRUE, "代码"=3, "source"=""} ("error out") T3 {"status"=TRUE, "代码"=3, "source"=""} ("error out") T3 {"status"=TRUE, "代码"=3, "source"=""} ("error out") T3 {"status"=TRUE, "代码"=3, "source"=""} ("error out") T3 {"status"=TRUE, "代码"=3, "source"=""} ("error out") T3 {"status"=TRUE, "代码"=3, "source"=""} ("error out") T3 {"status"=TRUE, "代码"=3, "source"=""} ("error out") T3 {"status"=TRUE, "代码"=3, "source"=""} ("error out") T3 {"status"=TRUE, "代码"=3, "source"=""} ("error out") T3 {"status"=TRUE, "代码"=3, "source"=""} ("error out")] -> w714
        frame "", Default {
        }
        frame "CODMn" {
        }
        frame "PH" {
        }
        frame "氨氮" {
        }
        frame "总氮" {
        }
        frame "总磷" {
        }
        frame "CODCr" {
        }
        frame "电导率" {
        }
        frame "水温" {
        }
        frame "溶解氧" {
        }
        frame "浊度" {
        }
        frame "叶绿素" {
        }
        frame "藻密度" {
        }
        frame "ORP" {
        }
      }
    }
    frame "i13102" {
      # "F1/ORPB"
      n87 = property class="Enum (严格)"(reference=w745) -> ("RingText.Text"=w749:string)  [unwired: 1 in, 2 out]
      n88 = case shown="\"\", 默认" w744 {
        tunnel: [FALSE TRUE TRUE TRUE TRUE TRUE TRUE TRUE TRUE TRUE TRUE TRUE TRUE TRUE] -> w747
        tunnel: [T3 {"status"=TRUE, "代码"=3, "source"=""} ("error out") T3 {"status"=TRUE, "代码"=3, "source"=""} ("error out") T3 {"status"=TRUE, "代码"=3, "source"=""} ("error out") T3 {"status"=TRUE, "代码"=3, "source"=""} ("error out") T3 {"status"=TRUE, "代码"=3, "source"=""} ("error out") T3 {"status"=TRUE, "代码"=3, "source"=""} ("error out") T3 {"status"=TRUE, "代码"=3, "source"=""} ("error out") T3 {"status"=TRUE, "代码"=3, "source"=""} ("error out") T3 {"status"=TRUE, "代码"=3, "source"=""} ("error out") T3 {"status"=TRUE, "代码"=3, "source"=""} ("error out") T3 {"status"=TRUE, "代码"=3, "source"=""} ("error out") T3 {"status"=TRUE, "代码"=3, "source"=""} ("error out") T3 {"status"=TRUE, "代码"=3, "source"=""} ("error out") T3 {"status"=TRUE, "代码"=3, "source"=""} ("error out")] -> w748
        frame "", Default {
        }
        frame "CODMn" {
        }
        frame "PH" {
        }
        frame "氨氮" {
        }
        frame "总氮" {
        }
        frame "总磷" {
        }
        frame "CODCr" {
        }
        frame "电导率" {
        }
        frame "水温" {
        }
        frame "溶解氧" {
        }
        frame "浊度" {
        }
        frame "叶绿素" {
        }
        frame "藻密度" {
        }
        frame "ORP" {
        }
      }
    }
    frame "i13103" {
      # "F2/ORPK"
      n89 = property class="Enum (严格)"(reference=w779) -> ("RingText.Text"=w783:string)  [unwired: 1 in, 2 out]
      n90 = case shown="\"\", 默认" w778 {
        tunnel: [FALSE TRUE TRUE TRUE TRUE TRUE TRUE TRUE TRUE TRUE TRUE TRUE TRUE TRUE] -> w781
        tunnel: [T3 {"status"=TRUE, "代码"=3, "source"=""} ("error out") T3 {"status"=TRUE, "代码"=3, "source"=""} ("error out") T3 {"status"=TRUE, "代码"=3, "source"=""} ("error out") T3 {"status"=TRUE, "代码"=3, "source"=""} ("error out") T3 {"status"=TRUE, "代码"=3, "source"=""} ("error out") T3 {"status"=TRUE, "代码"=3, "source"=""} ("error out") T3 {"status"=TRUE, "代码"=3, "source"=""} ("error out") T3 {"status"=TRUE, "代码"=3, "source"=""} ("error out") T3 {"status"=TRUE, "代码"=3, "source"=""} ("error out") T3 {"status"=TRUE, "代码"=3, "source"=""} ("error out") T3 {"status"=TRUE, "代码"=3, "source"=""} ("error out") T3 {"status"=TRUE, "代码"=3, "source"=""} ("error out") T3 {"status"=TRUE, "代码"=3, "source"=""} ("error out") T3 {"status"=TRUE, "代码"=3, "source"=""} ("error out")] -> w782
        frame "", Default {
        }
        frame "CODMn" {
        }
        frame "PH" {
        }
        frame "氨氮" {
        }
        frame "总氮" {
        }
        frame "总磷" {
        }
        frame "CODCr" {
        }
        frame "电导率" {
        }
        frame "水温" {
        }
        frame "溶解氧" {
        }
        frame "浊度" {
        }
        frame "叶绿素" {
        }
        frame "藻密度" {
        }
        frame "ORP" {
        }
      }
    }
    frame "i13104" {
      # "F3"
      n91 = property class="Enum (严格)"(reference=w817) -> ("RingText.Text"=w815:string)  [unwired: 1 in, 2 out]
      n92 = case shown="\"\", 默认" w816 {
        tunnel: [FALSE TRUE TRUE TRUE TRUE TRUE TRUE TRUE TRUE TRUE TRUE TRUE TRUE TRUE] -> w813
        tunnel: [T3 {"status"=TRUE, "代码"=3, "source"=""} ("error out") T3 {"status"=TRUE, "代码"=3, "source"=""} ("error out") T3 {"status"=TRUE, "代码"=3, "source"=""} ("error out") T3 {"status"=TRUE, "代码"=3, "source"=""} ("error out") T3 {"status"=TRUE, "代码"=3, "source"=""} ("error out") T3 {"status"=TRUE, "代码"=3, "source"=""} ("error out") T3 {"status"=TRUE, "代码"=3, "source"=""} ("error out") T3 {"status"=TRUE, "代码"=3, "source"=""} ("error out") T3 {"status"=TRUE, "代码"=3, "source"=""} ("error out") T3 {"status"=TRUE, "代码"=3, "source"=""} ("error out") T3 {"status"=TRUE, "代码"=3, "source"=""} ("error out") T3 {"status"=TRUE, "代码"=3, "source"=""} ("error out") T3 {"status"=TRUE, "代码"=3, "source"=""} ("error out") T3 {"status"=TRUE, "代码"=3, "source"=""} ("error out")] -> w814
        frame "", Default {
        }
        frame "CODMn" {
        }
        frame "PH" {
        }
        frame "氨氮" {
        }
        frame "总氮" {
        }
        frame "总磷" {
        }
        frame "CODCr" {
        }
        frame "电导率" {
        }
        frame "水温" {
        }
        frame "溶解氧" {
        }
        frame "浊度" {
        }
        frame "叶绿素" {
        }
        frame "藻密度" {
        }
        frame "ORP" {
        }
      }
    }
    frame "i13105" {
      # "F4"
      n93 = property class="Enum (严格)"(reference=w847) -> ("RingText.Text"=w851:string)  [unwired: 1 in, 2 out]
      n94 = case shown="\"\", 默认" w846 {
        tunnel: [FALSE TRUE TRUE TRUE TRUE TRUE TRUE TRUE TRUE TRUE TRUE TRUE TRUE TRUE] -> w849
        tunnel: [T3 {"status"=TRUE, "代码"=3, "source"=""} ("error out") T3 {"status"=TRUE, "代码"=3, "source"=""} ("error out") T3 {"status"=TRUE, "代码"=3, "source"=""} ("error out") T3 {"status"=TRUE, "代码"=3, "source"=""} ("error out") T3 {"status"=TRUE, "代码"=3, "source"=""} ("error out") T3 {"status"=TRUE, "代码"=3, "source"=""} ("error out") T3 {"status"=TRUE, "代码"=3, "source"=""} ("error out") T3 {"status"=TRUE, "代码"=3, "source"=""} ("error out") T3 {"status"=TRUE, "代码"=3, "source"=""} ("error out") T3 {"status"=TRUE, "代码"=3, "source"=""} ("error out") T3 {"status"=TRUE, "代码"=3, "source"=""} ("error out") T3 {"status"=TRUE, "代码"=3, "source"=""} ("error out") T3 {"status"=TRUE, "代码"=3, "source"=""} ("error out") T3 {"status"=TRUE, "代码"=3, "source"=""} ("error out")] -> w850
        frame "", Default {
        }
        frame "CODMn" {
        }
        frame "PH" {
        }
        frame "氨氮" {
        }
        frame "总氮" {
        }
        frame "总磷" {
        }
        frame "CODCr" {
        }
        frame "电导率" {
        }
        frame "水温" {
        }
        frame "溶解氧" {
        }
        frame "浊度" {
        }
        frame "叶绿素" {
        }
        frame "藻密度" {
        }
        frame "ORP" {
        }
      }
    }
    frame "i13106" {
      # "F5"
      n95 = property class="Enum (严格)"(reference=w881) -> ("RingText.Text"=w885:string)  [unwired: 1 in, 2 out]
      n96 = case shown="\"\", 默认" w880 {
        tunnel: [FALSE TRUE TRUE TRUE TRUE TRUE TRUE TRUE TRUE TRUE TRUE TRUE TRUE TRUE] -> w883
        tunnel: [T3 {"status"=TRUE, "代码"=3, "source"=""} ("error out") T3 {"status"=TRUE, "代码"=3, "source"=""} ("error out") T3 {"status"=TRUE, "代码"=3, "source"=""} ("error out") T3 {"status"=TRUE, "代码"=3, "source"=""} ("error out") T3 {"status"=TRUE, "代码"=3, "source"=""} ("error out") T3 {"status"=TRUE, "代码"=3, "source"=""} ("error out") T3 {"status"=TRUE, "代码"=3, "source"=""} ("error out") T3 {"status"=TRUE, "代码"=3, "source"=""} ("error out") T3 {"status"=TRUE, "代码"=3, "source"=""} ("error out") T3 {"status"=TRUE, "代码"=3, "source"=""} ("error out") T3 {"status"=TRUE, "代码"=3, "source"=""} ("error out") T3 {"status"=TRUE, "代码"=3, "source"=""} ("error out") T3 {"status"=TRUE, "代码"=3, "source"=""} ("error out") T3 {"status"=TRUE, "代码"=3, "source"=""} ("error out")] -> w884
        frame "", Default {
        }
        frame "CODMn" {
        }
        frame "PH" {
        }
        frame "氨氮" {
        }
        frame "总氮" {
        }
        frame "总磷" {
        }
        frame "CODCr" {
        }
        frame "电导率" {
        }
        frame "水温" {
        }
        frame "溶解氧" {
        }
        frame "浊度" {
        }
        frame "叶绿素" {
        }
        frame "藻密度" {
        }
        frame "ORP" {
        }
      }
    }
    frame "i13107" {
      # "F6"
      n97 = property class="Enum (严格)"(reference=w915) -> ("RingText.Text"=w919:string)  [unwired: 1 in, 2 out]
      n98 = case shown="\"\", 默认" w914 {
        tunnel: [FALSE TRUE TRUE TRUE TRUE TRUE TRUE TRUE TRUE TRUE TRUE TRUE TRUE TRUE] -> w917
        tunnel: [T3 {"status"=TRUE, "代码"=3, "source"=""} ("error out") T3 {"status"=TRUE, "代码"=3, "source"=""} ("error out") T3 {"status"=TRUE, "代码"=3, "source"=""} ("error out") T3 {"status"=TRUE, "代码"=3, "source"=""} ("error out") T3 {"status"=TRUE, "代码"=3, "source"=""} ("error out") T3 {"status"=TRUE, "代码"=3, "source"=""} ("error out") T3 {"status"=TRUE, "代码"=3, "source"=""} ("error out") T3 {"status"=TRUE, "代码"=3, "source"=""} ("error out") T3 {"status"=TRUE, "代码"=3, "source"=""} ("error out") T3 {"status"=TRUE, "代码"=3, "source"=""} ("error out") T3 {"status"=TRUE, "代码"=3, "source"=""} ("error out") T3 {"status"=TRUE, "代码"=3, "source"=""} ("error out") T3 {"status"=TRUE, "代码"=3, "source"=""} ("error out") T3 {"status"=TRUE, "代码"=3, "source"=""} ("error out")] -> w918
        frame "", Default {
        }
        frame "CODMn" {
        }
        frame "PH" {
        }
        frame "氨氮" {
        }
        frame "总氮" {
        }
        frame "总磷" {
        }
        frame "CODCr" {
        }
        frame "电导率" {
        }
        frame "水温" {
        }
        frame "溶解氧" {
        }
        frame "浊度" {
        }
        frame "叶绿素" {
        }
        frame "藻密度" {
        }
        frame "ORP" {
        }
      }
    }
    frame "i13108" {
      # "F7"
      n99 = property class="Enum (严格)"(reference=w949) -> ("RingText.Text"=w953:string)  [unwired: 1 in, 2 out]
      n100 = case shown="\"\", 默认" w948 {
        tunnel: [FALSE TRUE TRUE TRUE TRUE TRUE TRUE TRUE TRUE TRUE TRUE TRUE TRUE TRUE] -> w951
        tunnel: [T3 {"status"=TRUE, "代码"=3, "source"=""} ("error out") T3 {"status"=TRUE, "代码"=3, "source"=""} ("error out") T3 {"status"=TRUE, "代码"=3, "source"=""} ("error out") T3 {"status"=TRUE, "代码"=3, "source"=""} ("error out") T3 {"status"=TRUE, "代码"=3, "source"=""} ("error out") T3 {"status"=TRUE, "代码"=3, "source"=""} ("error out") T3 {"status"=TRUE, "代码"=3, "source"=""} ("error out") T3 {"status"=TRUE, "代码"=3, "source"=""} ("error out") T3 {"status"=TRUE, "代码"=3, "source"=""} ("error out") T3 {"status"=TRUE, "代码"=3, "source"=""} ("error out") T3 {"status"=TRUE, "代码"=3, "source"=""} ("error out") T3 {"status"=TRUE, "代码"=3, "source"=""} ("error out") T3 {"status"=TRUE, "代码"=3, "source"=""} ("error out") T3 {"status"=TRUE, "代码"=3, "source"=""} ("error out")] -> w952
        frame "", Default {
        }
        frame "CODMn" {
        }
        frame "PH" {
        }
        frame "氨氮" {
        }
        frame "总氮" {
        }
        frame "总磷" {
        }
        frame "CODCr" {
        }
        frame "电导率" {
        }
        frame "水温" {
        }
        frame "溶解氧" {
        }
        frame "浊度" {
        }
        frame "叶绿素" {
        }
        frame "藻密度" {
        }
        frame "ORP" {
        }
      }
    }
    frame "i13109" {
      # "X0/滴定数"
      n101 = property class="Enum (严格)"(reference=w983) -> ("RingText.Text"=w987:string)  [unwired: 1 in, 2 out]
      n102 = case shown="\"\", 默认" w982 {
        tunnel: [FALSE TRUE TRUE TRUE TRUE TRUE TRUE TRUE TRUE TRUE TRUE TRUE TRUE TRUE] -> w985
        tunnel: [T3 {"status"=TRUE, "代码"=3, "source"=""} ("error out") T3 {"status"=TRUE, "代码"=3, "source"=""} ("error out") T3 {"status"=TRUE, "代码"=3, "source"=""} ("error out") T3 {"status"=TRUE, "代码"=3, "source"=""} ("error out") T3 {"status"=TRUE, "代码"=3, "source"=""} ("error out") T3 {"status"=TRUE, "代码"=3, "source"=""} ("error out") T3 {"status"=TRUE, "代码"=3, "source"=""} ("error out") T3 {"status"=TRUE, "代码"=3, "source"=""} ("error out") T3 {"status"=TRUE, "代码"=3, "source"=""} ("error out") T3 {"status"=TRUE, "代码"=3, "source"=""} ("error out") T3 {"status"=TRUE, "代码"=3, "source"=""} ("error out") T3 {"status"=TRUE, "代码"=3, "source"=""} ("error out") T3 {"status"=TRUE, "代码"=3, "source"=""} ("error out") T3 {"status"=TRUE, "代码"=3, "source"=""} ("error out")] -> w986
        frame "", Default {
        }
        frame "CODMn" {
        }
        frame "PH" {
        }
        frame "氨氮" {
        }
        frame "总氮" {
        }
        frame "总磷" {
        }
        frame "CODCr" {
        }
        frame "电导率" {
        }
        frame "水温" {
        }
        frame "溶解氧" {
        }
        frame "浊度" {
        }
        frame "叶绿素" {
        }
        frame "藻密度" {
        }
        frame "ORP" {
        }
      }
    }
    frame "i13110" {
      # "量程"
      n103 = property class="Enum (严格)"(reference=w1017) -> ("RingText.Text"=w1021:string)  [unwired: 1 in, 2 out]
      n104 = case shown="\"\", 默认" w1016 {
        tunnel: [FALSE TRUE TRUE TRUE TRUE TRUE TRUE TRUE TRUE TRUE TRUE TRUE TRUE TRUE] -> w1019
        tunnel: [T3 {"status"=TRUE, "代码"=3, "source"=""} ("error out") T3 {"status"=TRUE, "代码"=3, "source"=""} ("error out") T3 {"status"=TRUE, "代码"=3, "source"=""} ("error out") T3 {"status"=TRUE, "代码"=3, "source"=""} ("error out") T3 {"status"=TRUE, "代码"=3, "source"=""} ("error out") T3 {"status"=TRUE, "代码"=3, "source"=""} ("error out") T3 {"status"=TRUE, "代码"=3, "source"=""} ("error out") T3 {"status"=TRUE, "代码"=3, "source"=""} ("error out") T3 {"status"=TRUE, "代码"=3, "source"=""} ("error out") T3 {"status"=TRUE, "代码"=3, "source"=""} ("error out") T3 {"status"=TRUE, "代码"=3, "source"=""} ("error out") T3 {"status"=TRUE, "代码"=3, "source"=""} ("error out") T3 {"status"=TRUE, "代码"=3, "source"=""} ("error out") T3 {"status"=TRUE, "代码"=3, "source"=""} ("error out")] -> w1020
        frame "", Default {
        }
        frame "CODMn" {
        }
        frame "PH" {
        }
        frame "氨氮" {
        }
        frame "总氮" {
        }
        frame "总磷" {
        }
        frame "CODCr" {
        }
        frame "电导率" {
        }
        frame "水温" {
        }
        frame "溶解氧" {
        }
        frame "浊度" {
        }
        frame "叶绿素" {
        }
        frame "藻密度" {
        }
        frame "ORP" {
        }
      }
    }
  }
  n105 = case shown="真" w8 {
    tunnel: w6 -> [_ w1052]
    tunnel: w5 -> [_ w1051]
    tunnel: w4 -> [_ w1050]
    frame False {
    }
    frame True {
      n106 = call "执行结果反馈与日志存储.vi"("日志信息"=w1051, "error out"=w1050, "设备"=w1052) -> ()  [unwired: 9 in]
    }
  }
